vi "PIM Flatten Test Parameters.vi"(7 "Test Configuration (\"\")":string, 9 "error in (no error)":errorcluster, 10 "Parameter Variant":variant) -> (1 "error out":errorcluster, 2 "Parameter String":string)   [LabVIEW 2011]
uses:
  PIM Version.vi
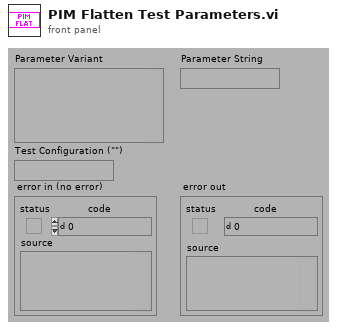
[diagram p1: front panel]
types:
  T1 = typedef "PIM Test Parameters.ctl" = cluster{"Stimulus":T2, "Measure":T4, "Display":T10}
  T2 = typedef "PIM Stimulus Parameters.ctl" = cluster{"C1 Pwr dBm":dbl, "C2 Pwr dBm":dbl, "Power Units":enum16{"dBm", "Watts"}, "Meas Type":enum32{"Time", "Frequency"}, "C1 Freq MHz":dbl, "C2 Freq MHz":dbl, "Swept Freq Step":T3}
  T3 = typedef "PIM Sweep Step Size.ctl" = u16
  T4 = typedef "PIM Measurement Parameters.ctl" = cluster{"IM Order":T5, "Direction":T6, "Averaging":T7, "ALC ON?":bool, "Peak Hold?":bool, "Peak last N":u32, "Ref Level dBm":dbl, "Ref Units":enum16{"dBm", "dBc"}, "Num Samples":u32, "Sample units":T8, "Update Rate (s)":dbl, "DUT PORT":T9, "Percent (%)":u8}
  T5 = typedef "IMOrder.ctl" = u8
  T6 = typedef "MeasMode.ctl" = u16
  T7 = typedef "HW Averaging.ctl" = u16
  T8 = typedef "PIM Meas Units.ctl" = enum16{"Sample(s)", "Second(s)", "Sweep(s)"}
  T9 = typedef "DUTport.ctl" = enum16{"Port 1", "Port 2"}
  T10 = typedef "PIM Display Parameters.ctl" = cluster{"Power Scale":cluster{"yRange_min":i32, "yRange_max":i32}, "xRange_span":u32}
  T11 = typedef "OGAB Version.ctl" = cluster{"Version":string, "Build Number":u32, "Build Date/Time":dbl}
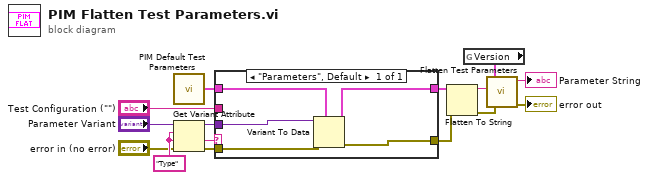
[diagram p0: block diagram]
diagram:
  w14 = "Type" ("name")
  n1 = call "PIM Default Test Parameters.vi"() -> ("Default PIM Test Parameters"=w1:T1)
  n2 = Get Variant Attribute(Variant="Parameter Variant", name=w14, default value (empty Variant)=w14, error in="error in (no error)") -> (duplicate Variant=w5:variant, value=w4:string, error out=w6:errorcluster)  [unwired: 1 out]
  n3 = case shown="\"Parameters\", Default" w4 {
    tunnel: w5 -> [w20]
    tunnel: w1 -> [w16]
    tunnel: [w17] -> w2
    tunnel: [w19] -> w3
    tunnel: w6 -> [w18]
    tunnel: "Test Configuration (\"\")" -> [_]
    frame "Parameters", Default {
      n4 = Variant To Data(error in=w18, type=w16, Variant=w20) -> (data=w17:T1, error out=w19:errorcluster)
    }
  }
  n5 = Flatten To String(anything=w2, error in (no error)=w3) -> (data string=w13:string, error out=w11:errorcluster)  [unwired: 3 out]
  n6 = global read "PIM Version.vi" "Version"() -> (w12:T11)
  n7 = call "Flatten Test Parameters.vi"("error in (no error)"=w11, "Flattened Test Parameters (\"\")"=w13, "Test Version"=w12) -> ("error out"=→"error out":errorcluster, "Flattened Test Parameters with Version"=→"Parameter String":string)  [unwired: 3 out]
